vi "msec sleep.vi"(8 "error in (no error)":errorcluster, 11 "msec":u32) -> (0 "error out":errorcluster)   [LabVIEW 2012, in "libximc.lvlib"]
doc: "void XIMC_API msec_sleep (unsigned int msec);"
uses:
  libximc.lvlib
  libximc.dll
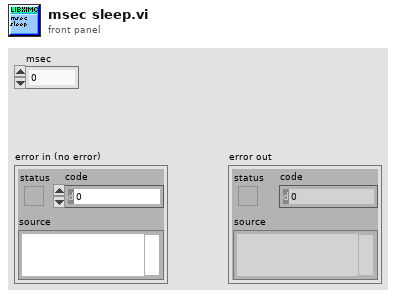
[diagram p1: front panel]
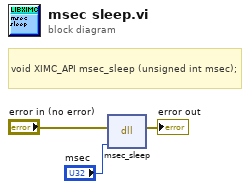
[diagram p0: block diagram]
diagram:
  # "void XIMC_API msec_sleep (unsigned int msec);"
  n1 = dll-call lib="E:/labview-2.12.1-Labview_12.0/ximcLVx32/libximc.*" fn="msec_sleep"(error in="error in (no error)", "msec"="msec") -> (error out=→"error out":errorcluster)  [unwired: 4 in, 1 out]
